vi "calc_scan_infos.vi"(8 "error in":errorcluster, 11 "All scan parameters":T2={"Fiber parameters"={"Frequency"=100.0, "Amplitude X"=0.0, "Amplitude Y"=0.0, "Initial Amplitude X"=0.0, "Initial Amplitude Y"=0.0, "Phase"=0.0}, "Spiral parameters"={"Imaging periods"=1.0, "Settling periods"=1.0, "Resting periods"=1.0}, "Run parameters"={"Run mode"=enum."Continuous", "Averages per frame"=1, "No. of frames"=1}, "Acquisition parameters"={"Cycles per pixel"=1, "Image size"=128}, "Fiber parameters pixel_mapper"={"Frequency"=1.0, "Amplitude X"=1.0, "Amplitude Y"=1.0, "Initial Amplitude X"=0.0, "Initial Amplitude Y"=0.0, "Phase"=0.0}, "Smooth_coeffs_cluster"={"Coeff 1"=0.0, "Coeff 2"=0.0}, "Storage parameters"={"Autosave"=FALSE, "Path"=path ""}} {"Smooth_coeffs_cluster"."Coeff 1" min=0.0 max=1.0 step=0.05; "Smooth_coeffs_cluster"."Coeff 2" min=0.0 max=1.0 step=0.05; "Fiber parameters pixel_mapper"."Phase" min=-90.0 max=90.0 step=5.0; "Fiber parameters pixel_mapper"."Initial Amplitude Y" min=0.0 max=1.0 step=0.1; "Fiber parameters pixel_mapper"."Initial Amplitude X" min=0.0 max=1.0 step=0.1; "Fiber parameters pixel_mapper"."Amplitude Y" min=0.0 max=3.0 step=0.1; "Fiber parameters pixel_mapper"."Amplitude X" min=0.0 max=3.0 step=0.1; "Fiber parameters pixel_mapper"."Frequency" min=100.0 max=6000.0 step=1.0; "Acquisition parameters"."Image size" items=["128x128 px"=128, "256x256 px"=256, "512x512 px"=512]; "Acquisition parameters"."Cycles per pixel" min=100 max=90000 step=1; "Run parameters"."No. of frames" min=1 max=1000 step=1; "Run parameters"."Averages per frame" min=1 max=32; "Spiral parameters"."Resting periods" min=10.0 max=1000.0 step=1.0; "Spiral parameters"."Settling periods" min=1.0 max=1000.0 step=1.0; "Spiral parameters"."Imaging periods" min=1.0 max=1000.0 step=1.0; "Fiber parameters"."Phase" min=-90.0 max=90.0 step=5.0; "Fiber parameters"."Initial Amplitude Y" min=0.0 max=1.0 step=0.1; "Fiber parameters"."Initial Amplitude X" min=0.0 max=1.0 step=0.1; "Fiber parameters"."Amplitude Y" min=0.0 max=3.0 step=0.1; "Fiber parameters"."Amplitude X" min=0.0 max=3.0 step=0.1; "Fiber parameters"."Frequency" min=100.0 max=6000.0 step=1.0}) -> (0 "error out":errorcluster, 3 "Scan infos":T1 {"Scan vs. Non-scan" scale=0.0..1.0})   [LabVIEW 2011, in "Fiberscope_library.lvlib"]
uses:
  Fiberscope_library.lvlib
  typedefs/all_scan_parameters_cluster.ctl
  typedefs/fiber_parameters_cluster.ctl
  typedefs/spiral_parameters_cluster.ctl
  typedefs/run_parameters_cluster.ctl
  typedefs/run_mode_enum.ctl
  typedefs/acquisition_parameters_cluster.ctl
  typedefs/image_size_I32.ctl
  typedefs/smooth_coeffs_cluster.ctl
  typedefs/storage_parameters_cluster.ctl
  typedefs/scan_infos.ctl
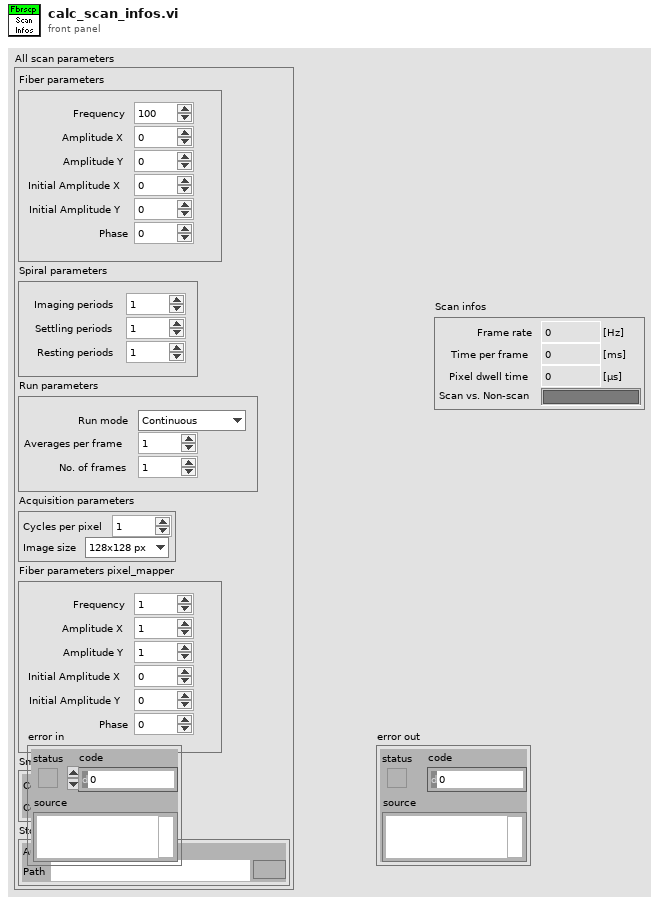
[diagram p1: front panel]
types:
  T1 = typedef "Fiberscope_library.lvlib/scan_infos.ctl" = cluster{"Frame rate":dbl, "Pixel dwell time":dbl, "Scan vs. Non-scan":dbl, "Time per frame":dbl}
  T2 = typedef "Fiberscope_library.lvlib/all_scan_parameters_cluster.ctl" = cluster{"Fiber parameters":T3, "Spiral parameters":T4, "Run parameters":T5, "Acquisition parameters":T7, "Fiber parameters pixel_mapper":T3, "Smooth_coeffs_cluster":T9, "Storage parameters":T10}
  T3 = typedef "Fiberscope_library.lvlib/fiber_parameters_cluster.ctl" = cluster{"Frequency":dbl, "Amplitude X":dbl, "Amplitude Y":dbl, "Initial Amplitude X":dbl, "Initial Amplitude Y":dbl, "Phase":dbl}
  T4 = typedef "Fiberscope_library.lvlib/spiral_parameters_cluster.ctl" = cluster{"Imaging periods":dbl, "Settling periods":dbl, "Resting periods":dbl}
  T5 = typedef "Fiberscope_library.lvlib/run_parameters_cluster.ctl" = cluster{"Run mode":T6, "Averages per frame":u8, "No. of frames":u32}
  T6 = typedef "Fiberscope_library.lvlib/run_mode_enum.ctl" = enum16{"Continuous", "Single frame", "No. of frames"}
  T7 = typedef "Fiberscope_library.lvlib/acquisition_parameters_cluster.ctl" = cluster{"Cycles per pixel":u32, "Image size":T8}
  T8 = typedef "Fiberscope_library.lvlib/image_size_I32.ctl" = i32
  T9 = typedef "Fiberscope_library.lvlib/smooth_coeffs_cluster.ctl" = cluster{"Coeff 1":dbl, "Coeff 2":dbl}
  T10 = typedef "Fiberscope_library.lvlib/storage_parameters_cluster.ctl" = cluster{"Autosave":bool, "Path":path}
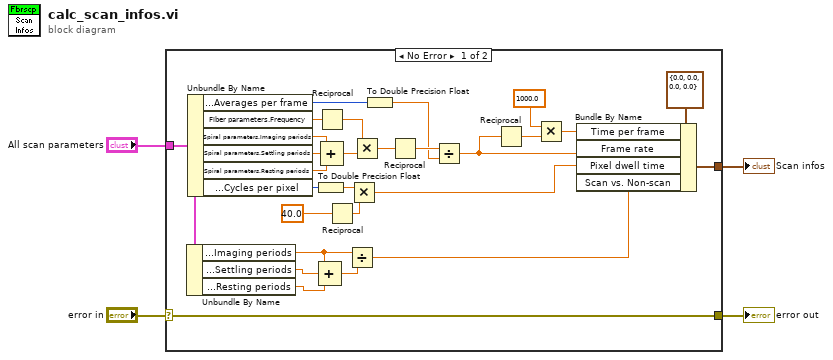
[diagram p0: block diagram]
diagram:
  n1 = case shown="No Error" "error in" {
    selector: "error in" -> [w32 w33]
    tunnel: [w32 w33] -> w3
    tunnel: "All scan parameters" -> [w17 _]
    tunnel: [w18 _] -> w1
    frame No Error {
      n2 = Unbundle By Name(w17) -> ("Spiral parameters.Imaging periods"=w12:dbl, "Spiral parameters.Settling periods"=w16:dbl, "Spiral parameters.Resting periods"=w15:dbl)
      n3 = Unbundle By Name(w17) -> ("Run parameters.Averages per frame"=w10:u8, "Fiber parameters.Frequency"=w31:dbl, "Spiral parameters.Imaging periods"=w30:dbl, "Spiral parameters.Settling periods"=w29:dbl, "Spiral parameters.Resting periods"=w28:dbl, "Acquisition parameters.Cycles per pixel"=w21:u32)
      n4 = To Double Precision Float(number=w21) -> (double precision float=w20:dbl)
      n5 = Reciprocal(x=w31) -> (1/x=w26:dbl)
      n6 = Compound Arithmetic op=ADD(w12, w16, w15) -> (w14:dbl)
      n7 = Compound Arithmetic op=ADD(w30, w29, w28) -> (w27:dbl)
      n8 = Reciprocal(x=40.0) -> (1/x=w23:dbl)
      n9 = Divide(x=w12, y=w14) -> (x/y=w13:dbl)
      n10 = Multiply(x=w20, y=w23) -> (x*y=w19:dbl)
      n11 = Multiply(x=w26, y=w27) -> (x*y=w25:dbl)
      n12 = To Double Precision Float(number=w10) -> (double precision float=w9:dbl)
      n13 = Reciprocal(x=w25) -> (1/x=w11:dbl)
      n14 = Divide(x=w11, y=w9) -> (x/y=w8:dbl)
      n15 = Reciprocal(x=w8) -> (1/x=w7:dbl)
      n16 = Multiply(x=1000.0, y=w7) -> (x*y=w5:dbl)
      n17 = Bundle By Name(cluster=T1 {"Frame rate"=0.0, "Pixel dwell time"=0.0, "Scan vs. Non-scan"=0.0, "Time per frame"=0.0} ("Scan infos"), "Time per frame"=w5, "Frame rate"=w8, "Pixel dwell time"=w19, "Scan vs. Non-scan"=w13) -> (w18:T1)
    }
    frame Error {
    }
  }
  "error out" <- w3
  "Scan infos" <- w1
